vi "Initialize.vi"(8 "error in (no error)":errorcluster, 10 "Stage Configuration":T1={"Serial Port"="COM4", "Forward Step (mm)"=0.4, "Lane Length (mm)"=6.0, "Lane Separation (mm)"=0.8, "Stage Type"=enum."Ti2", "Autofocus Z Planes"=9, "Autofocus Range (um)"=30.0, "Stage Limits"={"Y Min"=-4.5, "Y Max"=3.0, "X Min"=-19.0, "X Max"=33.5}, "Slide (mm)"={"top"=-13.0, "right"=-22.3, "width"=60.0, "height"=25.4}}) -> (0 "error out":errorcluster, 3 "Stage Controller out":refnum<class "Stage Controller.lvclass">)   [LabVIEW 2023, in "Stage Controller.lvlib" / "Stage Controller.lvclass"]
uses:
  Stage Controller.lvclass
  Resources/Type Defs/Stage Configuration.ctl
  Stage Controller.lvclass/Stage Controller.ctl
panel:
  out "Stage Configuration.Autofocus Range (um)":dbl
  in  "Stage Controller in":refnum<class "Stage Controller.lvclass">
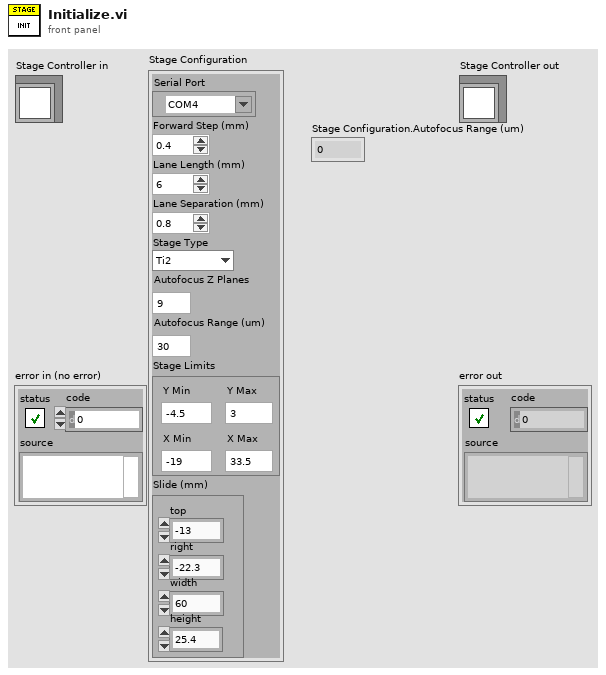
[diagram p1: front panel]
types:
  T1 = typedef "Stage Configuration.ctl" = cluster{"Serial Port":refnum<visa-resource-name>, "Forward Step (mm)":dbl, "Lane Length (mm)":dbl, "Lane Separation (mm)":dbl, "Stage Type":enum16{"Disabled", "ESP301", "Ti2", "Ludl", "ASI", "Simulate"}, "Autofocus Z Planes":i32, "Autofocus Range (um)":dbl, "Stage Limits":cluster{"Y Min":dbl, "Y Max":dbl, "X Min":dbl, "X Max":dbl}, "Slide (mm)":cluster{"top":dbl, "right":dbl, "width":dbl, "height":dbl}}
  T2 = enum16{"Disabled", "ESP301", "Ti2", "Ludl", "ASI", "Simulate"}
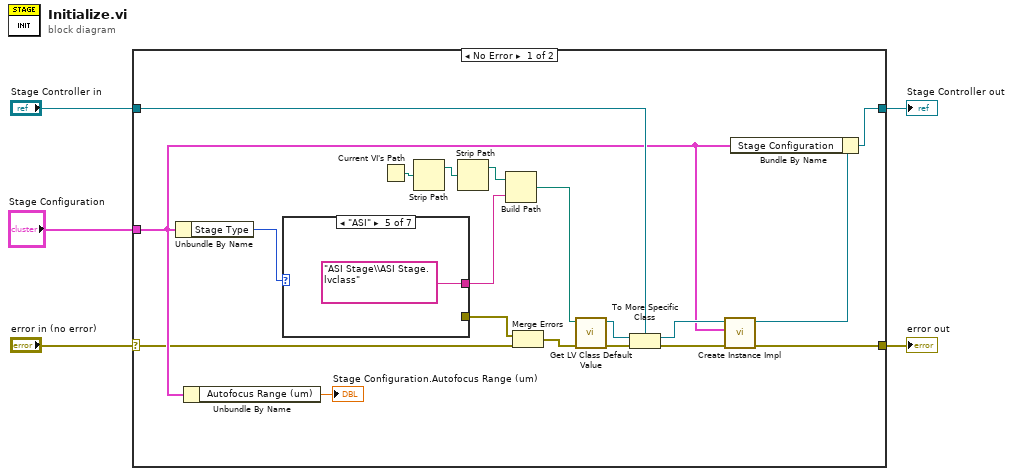
[diagram p0: block diagram]
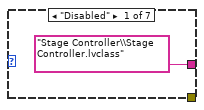
[diagram p2: hidden frame]
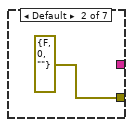
[diagram p3: hidden frame]
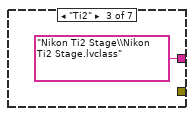
[diagram p4: hidden frame]
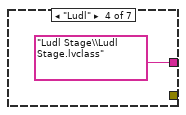
[diagram p5: hidden frame]
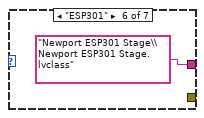
[diagram p6: hidden frame]
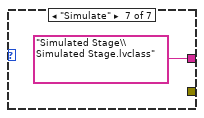
[diagram p7: hidden frame]
diagram:
  n1 = case shown="No Error" "error in (no error)" {
    selector: "error in (no error)" -> [w8 w33]
    tunnel: [w16 w33] -> w4
    tunnel: [w24 w32] -> w2
    tunnel: "Stage Controller in" -> [w14 w32]
    tunnel: "Stage Configuration" -> [w9 _]
    frame No Error {
      n2 = Unbundle By Name(w9) -> ("Stage Type"=w23:T2)
      n3 = Unbundle By Name(w9) -> ("Autofocus Range (um)"=→"Stage Configuration.Autofocus Range (um)":dbl)
      n4 = case shown="\"ASI\"" w23 {
        tunnel: ["Stage Controller\\Stage Controller.lvclass" _ "Nikon Ti2 Stage\\Nikon Ti2 Stage.lvclass" "Ludl Stage\\Ludl Stage.lvclass" "ASI Stage\\ASI Stage.lvclass" "Newport ESP301 Stage\\Newport ESP301 Stage.lvclass" "Simulated Stage\\Simulated Stage.lvclass"] -> w12
        tunnel: [_ errorcluster {"status"=FALSE, "code"=0, "source"=""} ("error IO") _ _ _ _ _] -> w6
        frame "Disabled" {
        }
        frame Default {
        }
        frame "Ti2" {
        }
        frame "Ludl" {
        }
        frame "ASI" {
        }
        frame "ESP301" {
        }
        frame "Simulate" {
        }
      }
      n5 = Current VI's Path() -> (path=w22:path)
      n6 = Strip Path(path=w22) -> (stripped path=w21:path)  [unwired: 1 out]
      n7 = Strip Path(path=w21) -> (stripped path=w20:path)  [unwired: 1 out]
      n8 = Build Path(base path=w20, name or relative path=w12) -> (appended path=w13:path)
      n9 = Merge Errors(w6, w8) -> (w7:errorcluster)
      n10 = call <vilib>:"Get LV Class Default Value.vi"("error in (no error)"=w7, "class path"=w13) -> ("error out"=w19:errorcluster, "object"=w18:refnum<class>)  [unwired: 8 in]
      n11 = To More Specific Class(target class=w14, reference=w18, error in=w19) -> (specific class reference=w11:refnum<class "Stage Controller.lvclass">, error out=w17:errorcluster)
      n12 = call-dynamic "Create Instance Impl.vi"("error in (no error)"=w17, "Stage Configuration"=w9, "Stage Controller in"=w11) -> ("error out"=w16:errorcluster, "Stage Controller out"=w15:refnum<class "Stage Controller.lvclass">)  [unwired: 7 in]
      n13 = Bundle By Name(cluster=w15, "Stage Configuration"=w9) -> (w24:refnum<class "Stage Controller.lvclass">)
    }
    frame Error {
    }
  }
  "error out" <- w4
  "Stage Controller out" <- w2
